vi "NI VeriStand - Close Waveform Session.vi"   [LabVIEW 2020, in "NI_VS Custom Device Waveform API.lvlib"]
doc: "Closes a waveform read or write session. Wire data to the <B>Single Waveform Read Session (DBL)</B> input to specify the instance to use."
uses:
  <vilib>/NI VeriStand/Custom Device Waveform API/NI_VS Custom Device Waveform API.lvlib
  <vilib>/NI VeriStand/Custom Device Waveform API/Multiple Waveforms Write (DBL)/Multiple Waveforms Write (DBL).lvclass
  <vilib>/NI VeriStand/Custom Device Waveform API/Single Waveform Read (DBL)/Single Waveform Read (DBL).lvclass
  <vilib>/NI VeriStand/Custom Device Waveform API/Single Waveform Read (CDB)/Single Waveform Read (CDB).lvclass
  <vilib>/NI VeriStand/Custom Device Waveform API/Multiple Waveforms Write (CDB)/Multiple Waveforms Write (CDB).lvclass
  <vilib>/NI VeriStand/Custom Device Waveform API/Multiple Waveforms Read (CDB)/Multiple Waveforms Read (CDB).lvclass
  <vilib>/NI VeriStand/Custom Device Waveform API/Multiple Waveforms Read (DBL)/Multiple Waveforms Read (DBL).lvclass
  <vilib>/NI VeriStand/Custom Device Waveform API/Single Waveform Write (DBL)/Single Waveform Write (DBL).lvclass
  <vilib>/NI VeriStand/Custom Device Waveform API/Single Waveform Write (CDB)/Single Waveform Write (CDB).lvclass
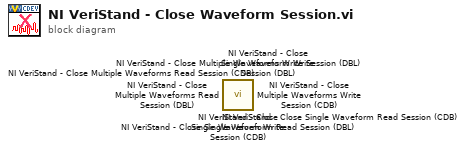
[diagram p0: block diagram]
diagram:
  n1 = call <vilib>:"NI VeriStand - Close Single Waveform Write Session (CDB).vi"() -> ()  [unwired: 11 in, 1 out]
  n2 = call <vilib>:"NI VeriStand - Close Single Waveform Write Session (DBL).vi"() -> ()  [unwired: 11 in, 1 out]
  n3 = call <vilib>:"NI VeriStand - Close Multiple Waveforms Read Session (DBL).vi"() -> ()  [unwired: 11 in, 1 out]
  n4 = call <vilib>:"NI VeriStand - Close Multiple Waveforms Write Session (CDB).vi"() -> ()  [unwired: 11 in, 1 out]
  n5 = call <vilib>:"NI VeriStand - Close Multiple Waveforms Read Session (CDB).vi"() -> ()  [unwired: 11 in, 1 out]
  n6 = call <vilib>:"NI VeriStand - Close Single Waveform Read Session (CDB).vi"() -> ()  [unwired: 11 in, 1 out]
  n7 = call <vilib>:"NI VeriStand - Close Single Waveform Read Session (DBL).vi"() -> ()  [unwired: 11 in, 1 out]
  n8 = call <vilib>:"NI VeriStand - Close Multiple Waveforms Write Session (DBL).vi"() -> ()  [unwired: 11 in, 1 out]
